vi "AlliGator Update Phasor Plot Image.vi"(4 "Compute Phasor Plot (T)":bool=TRUE, 5 "Phasor Plot Color Scale":refnum<vi>, 7 "Phasor Plot Display Range Refnum":refnum<vi>, 8 "error in (no error)":errorcluster, 9 "Corrected Complex Phasor Array":csg[][](array[numeric]), 11 "Phasor Plot Image in":T1) -> (0 "error out":errorcluster, 1 "Overlays":string[](array[string]), 3 "Phasor Plot Image out":T1)   [LabVIEW 2021, in "AlliGator Phasor Plot.lvlib"]
doc: "Updates the Phasor Plot image."
uses:
  AlliGator Phasor Plot.lvlib
  <vilib>/vision/Image Controls.llb/IMAQ Image.ctl
  Time/Time.lvlib
panel:
  out "CPU (s)":dbl
  # "see the AlliGator License on the block diagram (Ctrl+E or Window:Show Block Diagram)"
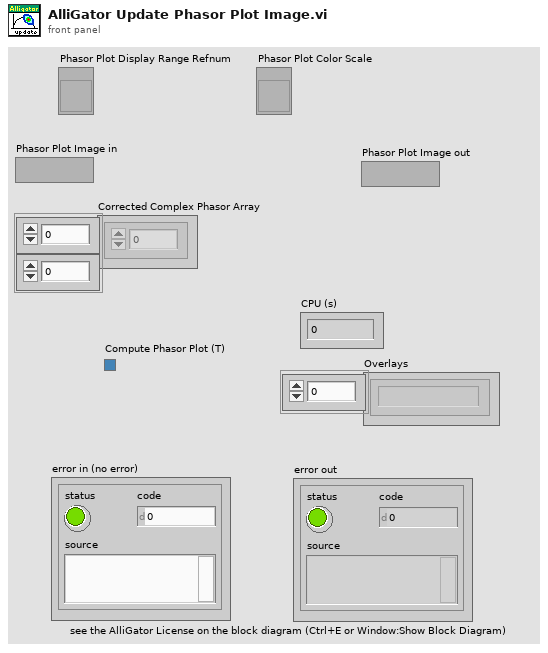
[diagram p1: front panel]
types:
  T1 = typedef "IMAQ Image.ctl" = refnum<image>
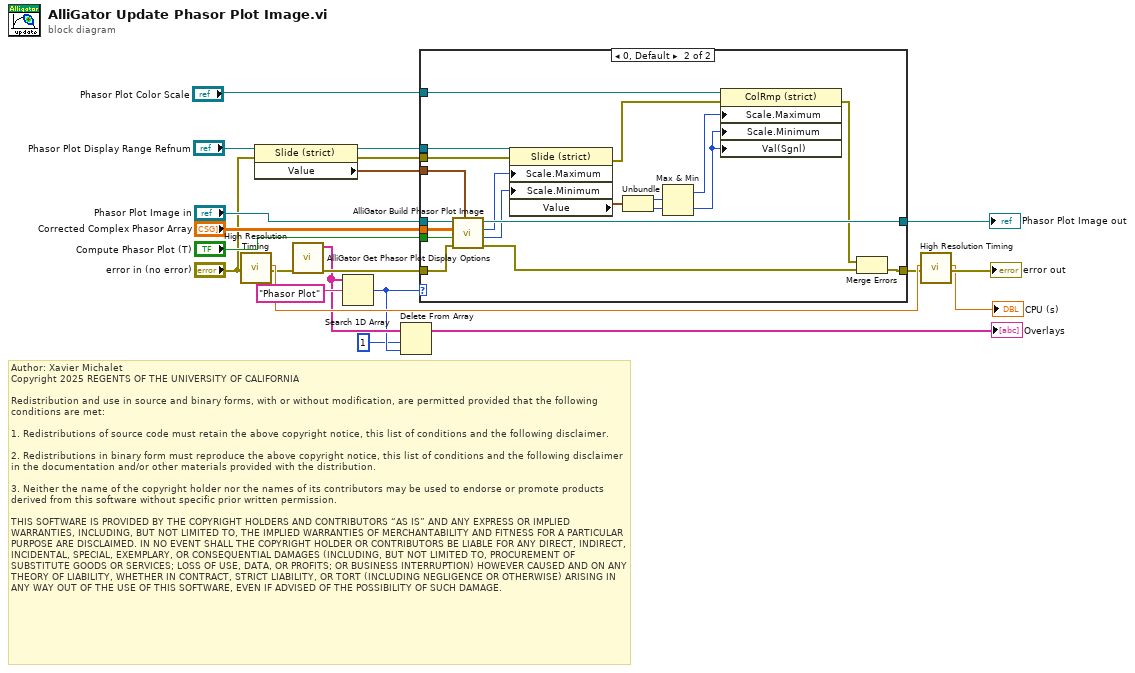
[diagram p0: block diagram]
diagram:
  # "Author: Xavier Michalet\nCopyright 2025 REGENTS OF THE UNIVERSITY OF CALIFORNIA\n\nRedistribution and use in source and binary forms, with or without modification, are permitted provided that the following conditions are met:\n\n1. Redistributions of source code must retain the above copyright notice, this list of conditions and the following disclaimer.\n\n2. Redistributions in binary form must reproduce the above copyright notice, this list of conditions and the following disclaimer in the documentation and/or other materials provided with the distribution.\n\n3. Neither the name of the copyright holder nor the names of its contributors may be used to endorse or promote products derived from this software without specific prior written permission.\n\nTHIS SOFTWARE IS PROVIDED BY THE COPYRIGHT HOLDERS AND CONTRIBUTORS “AS IS” AND ANY EXPRESS OR IMPLIED WARRANTIES, INCLUDING, BUT NOT LIMITED TO, THE IMPLIED WARRANTIES OF MERCHANTABILITY AND FITNESS FOR A PARTICULAR PURPOSE ARE DISCLAIMED. IN NO EVENT SHALL THE COPYRIGHT HOLDER OR CONTRIBUTORS BE LIABLE FOR ANY DIRECT, INDIRECT, INCIDENTAL, SPECIAL, EXEMPLARY, OR CONSEQUENTIAL DAMAGES (INCLUDING, BUT NOT LIMITED TO, PROCUREMENT OF SUBSTITUTE GOODS OR SERVICES; LOSS OF USE, DATA, OR PROFITS; OR BUSINESS INTERRUPTION) HOWEVER CAUSED AND ON ANY THEORY OF LIABILITY, WHETHER IN CONTRACT, STRICT LIABILITY, OR TORT (INCLUDING NEGLIGENCE OR OTHERWISE) ARISING IN ANY WAY OUT OF THE USE OF THIS SOFTWARE, EVEN IF ADVISED OF THE POSSIBILITY OF SUCH DAMAGE."
  n1 = call "High Resolution Timing.vi"("Error In"="error in (no error)") -> ("elapsed (relative) seconds"=w19:dbl, "Error Out"=w13:errorcluster)  [unwired: 16 in, 1 out]
  n2 = property class="Slide (strict)"(reference="Phasor Plot Display Range Refnum", error in="error in (no error)") -> (reference out=w3:refnum<vi>, error out=w2:errorcluster, "Value"=w4:cluster{u32, u32})
  n3 = call "AlliGator Get Phasor Plot Display Options.vi"("error in (no error)"=w13) -> ("error out"=w12:errorcluster, "Phasor Plot Image Elements to Update"=w10:string[])  [unwired: 9 in]
  n4 = Search 1D Array(1D array=w10, element="Phasor Plot") -> (index of element=w9:i32)  [unwired: 1 in]
  n5 = Delete From Array(array=w10, length=1, index=w9) -> (array with subset deleted=→"Overlays":string[])  [unwired: 1 out]
  n6 = case shown="0, Default" w9 {
    tunnel: "Corrected Complex Phasor Array" -> [_ w43]
    tunnel: "Phasor Plot Image in" -> [w23 w42]
    tunnel: w4 -> [_ w31]
    tunnel: [w23 w41] -> w18
    tunnel: [w22 w33] -> w17
    tunnel: "Compute Phasor Plot (T)" -> [_ w39]
    tunnel: w12 -> [w22 w38]
    tunnel: w3 -> [_ w35]
    tunnel: w2 -> [_ w34]
    tunnel: "Phasor Plot Color Scale" -> [_ w32]
    frame -1 {
    }
    frame 0, Default {
      n7 = call "AlliGator Build Phasor Plot Image.vi"("Display Range"=w31, "error in (no error)"=w38, "Compute Phasor Plot (T)"=w39, "Pixel Phasors Array (V x H)"=w43, "Phasor Plot Image in"=w42) -> ("error out"=w40:errorcluster, "min value"=w36:u32, "max value"=w37:u32, "Phasor Plot Image out"=w41:T1)  [unwired: 3 in]
      n8 = property class="Slide (strict)"(reference=w35, error in=w34, "Scale.Maximum"=w37, "Scale.Minimum"=w36) -> (error out=w29:errorcluster, "Value"=w28:cluster{u32, u32})  [unwired: 1 out]
      n9 = Unbundle(w28) -> (w27:u32, w26:u32)
      n10 = Max & Min(x=w27, y=w26) -> (max(x,y)=w25:u32, min(x,y)=w24:u32)
      n11 = property class="ColRmp (strict)"(reference=w32, error in=w29, "Scale.Maximum"=w25, "Scale.Minimum"=w24, "Val(Sgnl)"=w24) -> (error out=w30:errorcluster)  [unwired: 1 out]
      n12 = Merge Errors(w30, w40) -> (w33:errorcluster)
    }
  }
  "Phasor Plot Image out" <- w18
  n13 = call "High Resolution Timing.vi"("relative seconds (NaN)"=w19, "Error In"=w17) -> ("elapsed (relative) seconds"=→"CPU (s)":dbl, "Error Out"=→"error out":errorcluster)  [unwired: 15 in, 1 out]
